vi "Example_Single_Measurement_Tomography_v1.vi"() -> ()   [LabVIEW 2021]
uses:
  Ver_1/Config_File_Paths.ctl
panel:
  out "XY Graph 2":cluster{"Time":dbl[], "X":dbl[]}[](graph)
  out "Possible Mismatch In Phase (?)":bool
  out "Enough Points (?)":bool
  out "Trig Out Found(?)":bool
  out "XY Graph":cluster{"Time":dbl[], "X":dbl[]}[](graph)
  out "error out":errorcluster
  in  "Config files paths":T1={"ZI config file (.ini)"="Config_Ver_1\\Zurich_params.ini", "Keithley config file (.ini)"="Config_Ver_1\\Keithley_params.ini", "Arduino config file (.ini)"="Config_Ver_1\\pulse_sequence.ini"}
  in  "error in":errorcluster
  in  "Resource Address":T2={"ZI Address"="DEV714", "VISA Keithley"="", "VISA Arduino PG"=""}
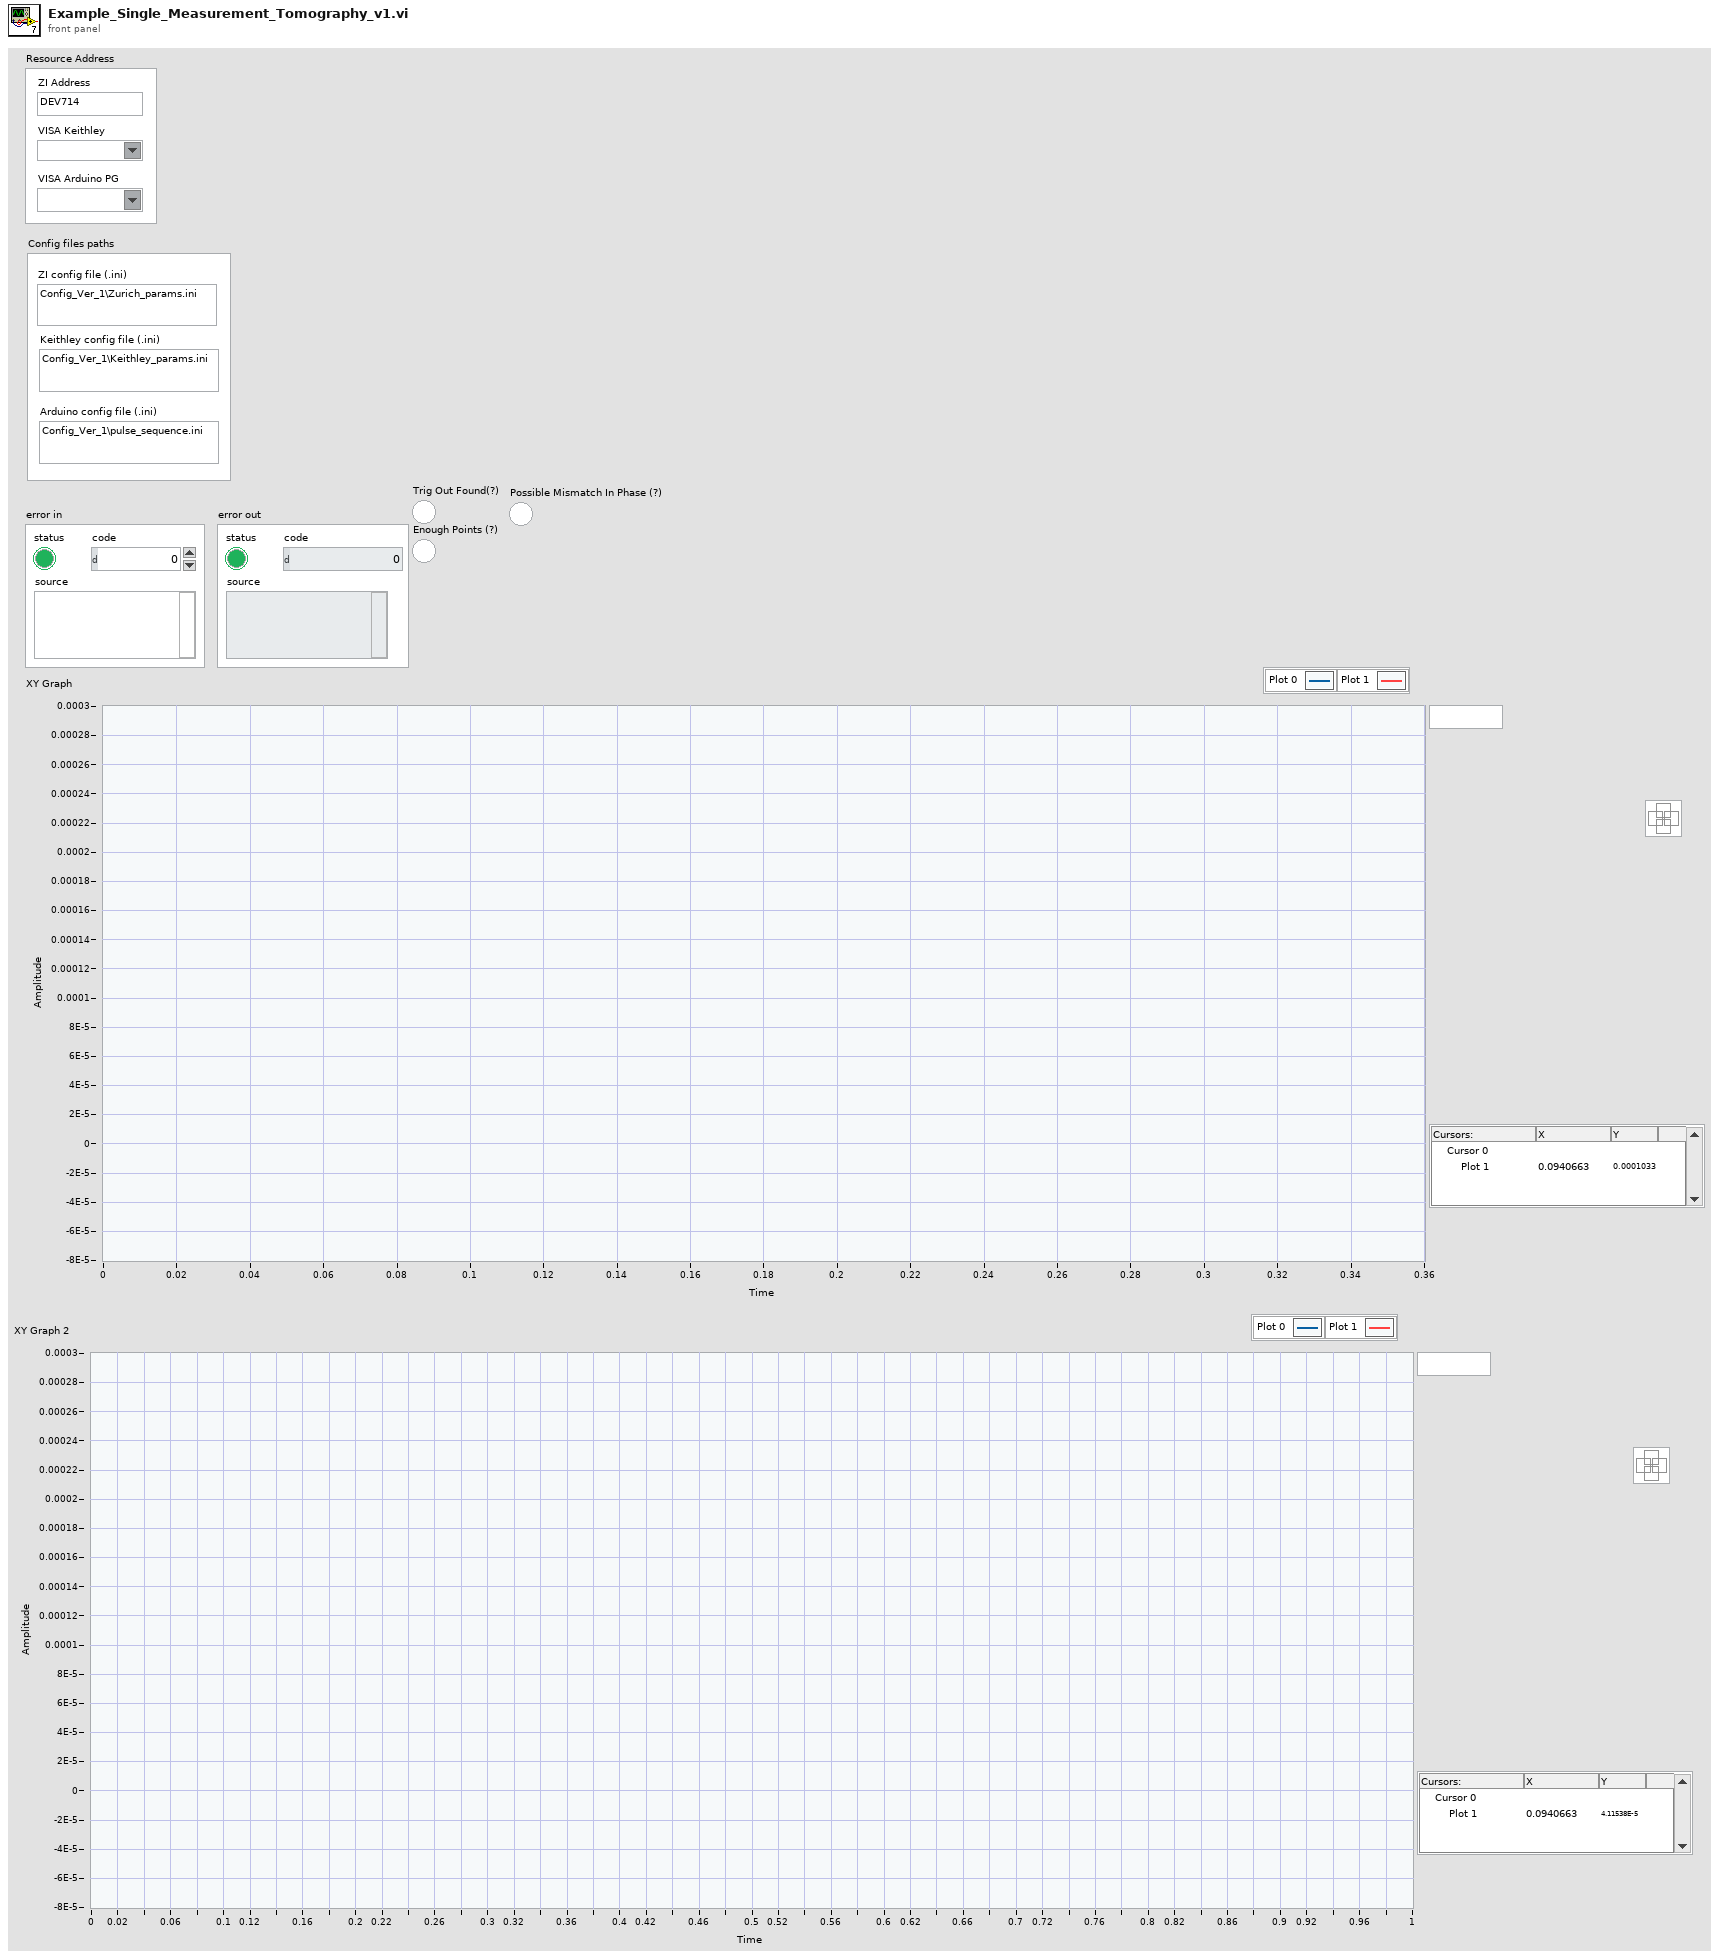
[diagram p1: front panel]
types:
  T1 = typedef "Config_File_Paths.ctl" = cluster{"ZI config file (.ini)":string, "Keithley config file (.ini)":string, "Arduino config file (.ini)":string}
  T2 = cluster{"ZI Address":string, "VISA Keithley":refnum<visa-resource-name>, "VISA Arduino PG":refnum<visa-resource-name>}
  T3 = typedef "Resources.ctl" = cluster{"ZI Handle":T4, "ZI ModHandle":T5, "VISA arduino":refnum<visa-resource-name>, "VISA Keithley":refnum<visa-resource-name>}
  T4 = typedef "Zurich Instruments LabOne.lvlib/ziTypeHandle.ctl" = cluster{"handleValid":bool, "Conn":u64, "Path Prefix":string, "Handle":u64, "Connected":bool, "Clockbase(s)":dbl}
  T5 = typedef "Zurich Instruments LabOne.lvlib/ziTypeModHandle.ctl" = cluster{"handleValid":bool, "Conn":u64, "ModHandle":u64, "moduleID":string, "Path Prefix":string}
  T6 = typedef "ZI_Data.ctl" = cluster{"R":dbl[], "Theta":dbl[], "X":dbl[], "Y":dbl[], "AuxIn0":dbl[], "AuxIn1":dbl[], "Frequency":dbl[], "DIO":dbl[], "Time":dbl[]}
  T7 = typedef "Cutted_Data.ctl" = cluster{"X":dbl[], "Y":dbl[], "Time":dbl[]}
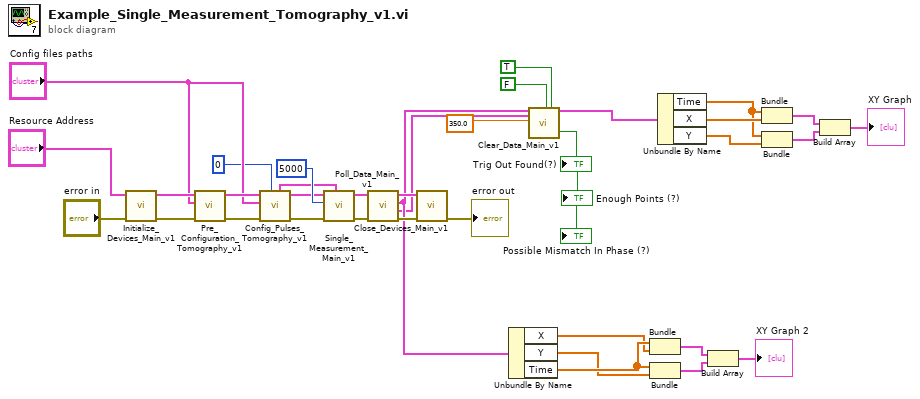
[diagram p0: block diagram]
diagram:
  n1 = call "Initialize_Devices_Main_v1.vi"("error in"="error in", "Resource Address"="Resource Address") -> ("error out"=w6:errorcluster, "Resources"=w5:T3)  [unwired: 8 in]
  n2 = call "Pre_Configuration_Tomography_v1.vi"("error in"=w6, "Config files paths"="Config files paths", "Resources in"=w5) -> ("error out"=w7:errorcluster, "Resources out"=w4:T3)  [unwired: 7 in]
  n3 = call "Config_Pulses_Tomography_v1.vi"("init file iterator"=u8 0, "error in"=w7, "Config files paths"="Config files paths", "Resources in"=w4) -> ("error out"=w8:errorcluster, "Resources out"=w9:T3, "Config files paths (single)"=w1:T1)  [unwired: 3 in, 2 out]
  n4 = call "Single_Measurement_Main_v1.vi"("Config files paths"=w1, "error in"=w8, "Timeout [ms]"=u64 5000, "Resources In"=w9) -> ("error out"=w34:errorcluster, "Resources Out"=w35:T3)  [unwired: 6 in]
  n5 = call "Poll_Data_Main_v1.vi"("error in"=w34, "Resources in"=w35) -> ("error out"=w32:errorcluster, "ZI Data 3"=w15:T6, "ZI Data 0"=w22:T6, "Resources out"=w33:T3)  [unwired: 6 in]
  n6 = call "Close_Devices_Main_v1.vi"("error in"=w32, "Resources in"=w33) -> ("error out"=→"error out":errorcluster)  [unwired: 9 in]
  n7 = Unbundle By Name(w22) -> ("X"=w17:dbl[], "Y"=w16:dbl[], "Time"=w18:dbl[])
  n8 = call "Clear_Data_Main_v1.vi"("ZI Data 0"=w22, "ZI Data 3"=w15, "Time Of Collected Data (ms)"=350.0, "Fixed Number Of Points"=FALSE, "Check Phase Mismatch"=TRUE) -> ("Trig Out Found(?)"=→"Trig Out Found(?)":bool, "Enough Points (?)"=→"Enough Points (?)":bool, "Possible Mismatch In Phase (?)"=→"Possible Mismatch In Phase (?)":bool, "Cutted Data"=w13:T7)  [unwired: 9 in, 2 out]
  n9 = Bundle("Time"=w18, "X"=w17) -> (w19:cluster{"Time":dbl[], "X":dbl[]})  [unwired: 1 in]
  n10 = Bundle("Time"=w18, "Y"=w16) -> (w20:cluster{"Time":dbl[], "Y":dbl[]})  [unwired: 1 in]
  n11 = Unbundle By Name(w13) -> ("Time"=w10:dbl[], "X"=w12:dbl[], "Y"=w11:dbl[])
  n12 = Build Array(w19, w20) -> (→"XY Graph 2":cluster{"Time":dbl[], "Y":dbl[]}[])
  n13 = Bundle("Time"=w10, "X"=w12) -> (w30:cluster{"Time":dbl[], "X":dbl[]})  [unwired: 1 in]
  n14 = Bundle("Time"=w10, "Y"=w11) -> (w29:cluster{"Time":dbl[], "Y":dbl[]})  [unwired: 1 in]
  n15 = Build Array(w30, w29) -> (→"XY Graph":cluster{"Time":dbl[], "Y":dbl[]}[])
